vi "Exit.vi"(8 "error in":errorcluster, 10 "Message Queues":T1, 11 "Notifiers":T2) -> (0 "error out":errorcluster)   [LabVIEW 2015, in "DAQ.lvlib"]
uses:
  Exercise/Production Line/DAQ/DAQ.lvlib
  Exercise/Production Line/support/Notifiers/Notifiers.ctl
  Exercise/Production Line/support/Message Queue/All Message Queues.ctl
  Exercise/Production Line/support/Message Queue/Message Cluster.ctl
  Exercise/Production Line/support/Message Queue/Enqueue Message (Single).vi
  Exercise/Production Line/support/Message Queue/Message Queue.lvlib
  Exercise/Production Line/support/Notifiers/Notifiers.lvlib
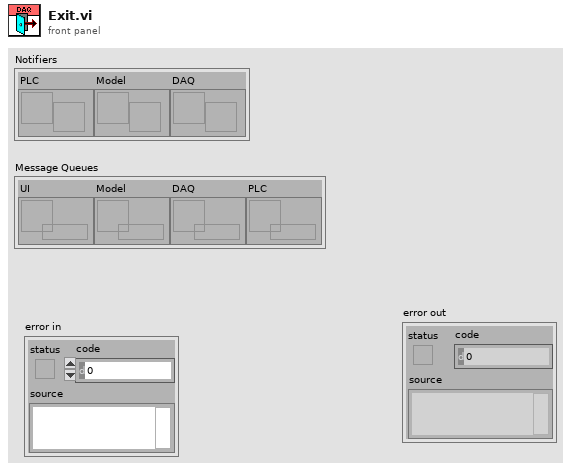
[diagram p1: front panel]
types:
  T1 = typedef "Message Queue.lvlib/All Message Queues.ctl" = cluster{"UI":refnum<queue>, "Model":refnum<queue>, "DAQ":refnum<queue>, "PLC":refnum<queue>}
  T2 = typedef "Notifiers.lvlib/Notifiers.ctl" = cluster{"PLC":refnum<notifier>, "Model":refnum<notifier>, "DAQ":refnum<notifier>}
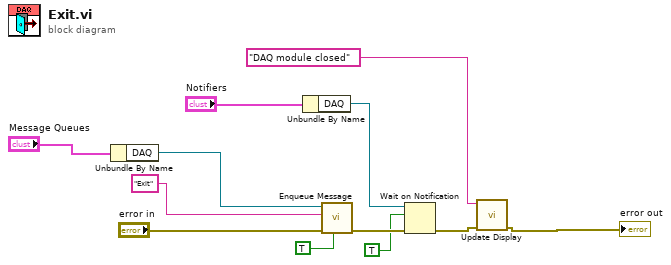
[diagram p0: block diagram]
diagram:
  n1 = Unbundle By Name("Message Queues") -> ("DAQ"=w5:refnum<queue>)
  n2 = Unbundle By Name("Notifiers") -> ("DAQ"=w6:refnum<notifier>)
  n3 = call-poly "Enqueue Message.vi"("Priority Message? (F)"=TRUE, "error in (no error)"="error in", "Message"="Exit", "Message Queue"=w5) -> ("error out"=w9:errorcluster)  [unwired: 6 in, 1 out]
  n4 = Wait on Notification(notifier=w6, ignore previous (F)=TRUE, error in (no error)=w9) -> (error out=w4:errorcluster)  [unwired: 1 in, 3 out]
  n5 = call "Update Display.vi"("error in"=w4, "Message string"="DAQ module closed" ("Message")) -> ("error out"=→"error out":errorcluster)  [unwired: 9 in]
